vi "Untitled 6 (SubVI).vi"(6 "Center coordinates (m)":cluster{"Xc":sgl, "Yc":sgl}, 7 "Size (m)":cluster{"Width":sgl, "Height":sgl}, 8 "error in (no error)":errorcluster, 9 "# of Grids":i32, 10 "Numeric":i32, 11 "Angle (deg)":sgl) -> (0 "error out":errorcluster, 3 "Array":sgl[][](array[numeric]))   [LabVIEW 2014]
panel:
  out "initialized array":dbl[][](array[numeric])
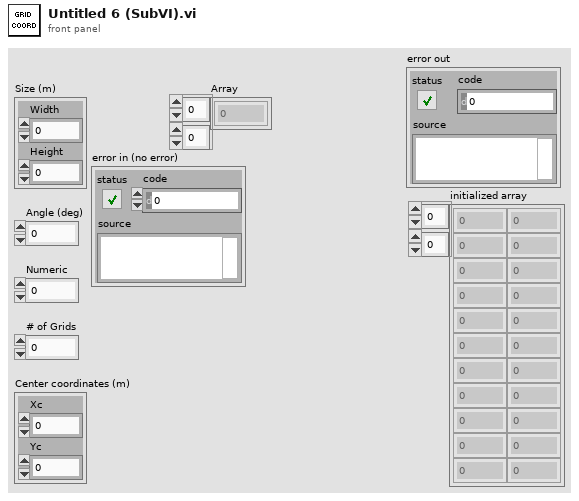
[diagram p1: front panel]
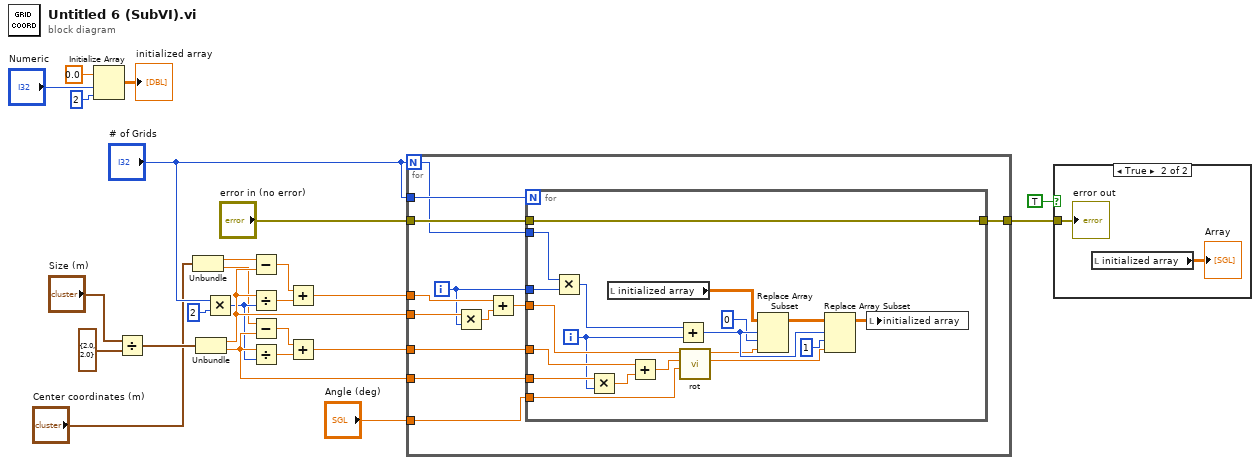
[diagram p0: block diagram]
diagram:
  n1 = Initialize Array(0.0 ("element"), "Numeric", 2 ("dimension size")) -> (→"initialized array":dbl[][])
  n2 = Divide(x="Size (m)", y=cluster{"Width":sgl, "Height":sgl} {"Width"=2.0, "Height"=2.0}) -> (x/y=w12:cluster{"Width":sgl, "Height":sgl})
  n3 = Unbundle("Center coordinates (m)") -> ("Xc"=w11:sgl, "Yc"=w13:sgl)
  n4 = Unbundle(w12) -> ("Width"=w24:sgl, "Height"=w23:sgl)
  n5 = Multiply(x="# of Grids", y=2) -> (x*y=w15:i32)
  n6 = Subtract(x=w11, y=w24) -> (x-y=w16:sgl)
  n7 = Divide(x=w24, y=w15) -> (x/y=w17:sgl)
  n8 = Subtract(x=w13, y=w23) -> (x-y=w18:sgl)
  n9 = Divide(x=w23, y=w15) -> (x/y=w19:sgl)
  n10 = Add(x=w16, y=w17) -> (x+y=w20:sgl)
  n11 = Add(x=w18, y=w19) -> (x+y=w22:sgl)
  n12 = for {
    N: "# of Grids" -> [w26]
    tunnel: w20 -> [w36]
    tunnel: w24 -> [w37]
    tunnel: "# of Grids" -> [w34]
    tunnel: w23 -> [w33]
    tunnel: w22 -> [w32]
    tunnel: "Angle (deg)" -> [w30]
    tunnel: [w29] -> w6
    tunnel: "error in (no error)" -> [w28]
    i -> [w27]
    n13 = Multiply(x=w37, y=w27) -> (x*y=w35:sgl)
    n14 = Add(x=w36, y=w35) -> (x+y=w31:sgl)
    n15 = for {
      N: w34 -> [_]
      tunnel: w33 -> [w56]
      tunnel: w32 -> [w54]
      tunnel: w31 -> [w53]
      tunnel: w30 -> [w51]
      tunnel: [w50] -> w29
      tunnel: w28 -> [w50]
      tunnel: w27 -> [w49]
      tunnel: w26 -> [w48]
      i -> [w46]
      n16 = Multiply(x=w48, y=w49) -> (x*y=w47:i32)
      n17 = Multiply(x=w56, y=w46) -> (x*y=w55:sgl)
      n18 = local read "initialized array"() -> (w43:dbl[][])
      n19 = Add(x=w54, y=w55) -> (x+y=w52:sgl)
      n20 = Add(x=w47, y=w46) -> (x+y=w45:i32)
      n21 = call "rot.vi"("angle"=w51, "y"=w52, "x"=w53) -> ("y'"=w39:sgl, "x'"=w40:sgl)  [unwired: 7 in]
      n22 = Replace Array Subset(array=w43, new element=w40, index (row)=w45, index (col)=0 ("disabled index (col)")) -> (w44:dbl[][])
      n23 = Replace Array Subset(array=w44, new element=w39, index (row)=w45, index (col)=1 ("disabled index (col)")) -> (w38:dbl[][])
      n24 = local write "initialized array"(w38) -> ()
    }
  }
  n25 = case shown="True" TRUE {
    tunnel: w6 -> [_ w58]
    frame False {
    }
    frame True {
      n26 = local read "initialized array"() -> (→"Array":dbl[][])
      "error out" <- w58
    }
  }
